vi "QCP Get.vi"   [LabVIEW 2015]
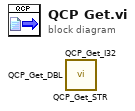
[diagram p0: block diagram]
diagram:
  n1 = call <userlib>:"QCP_Get_STR.vi"() -> ()  [unwired: 8 in, 3 out]
  n2 = call <userlib>:"QCP_Get_I32.vi"() -> ()  [unwired: 8 in, 3 out]
  n3 = call <userlib>:"QCP_Get_DBL.vi"() -> ()  [unwired: 8 in, 3 out]
